vi "Dband.vi"(9 "dband":dbl, 10 "Numeric":dbl) -> (2 "Fixed":dbl)   [LabVIEW 2020]
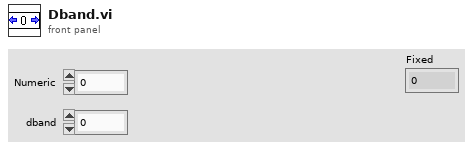
[diagram p1: front panel]
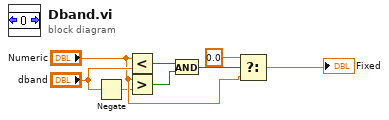
[diagram p0: block diagram]
diagram:
  n1 = Negate(x="dband") -> (-x=w1:dbl)
  n2 = Less?(x="Numeric", y="dband") -> (x < y?=w7:bool)
  n3 = Greater?(x="Numeric", y=w1) -> (0:w6:bool)
  n4 = And(x=w7, y=w6) -> (x .and. y?=w5:bool)
  n5 = Select(t=0.0, s=w5, f="Numeric") -> (s? t:f=→"Fixed":dbl)
